vi "EX PROJ - Rotating Laptop Stand.vi"() -> ()   [LabVIEW 2018]
uses:
  <vilib>/Analysis/baseanly.llb/Mean (DBL).vi
  <vilib>/Analysis/NI_AALBase.lvlib
panel:
  out "offset":dbl
  out "power":dbl
  out "picture":picture
  in  "stop 2":bool
  out "fps":dbl
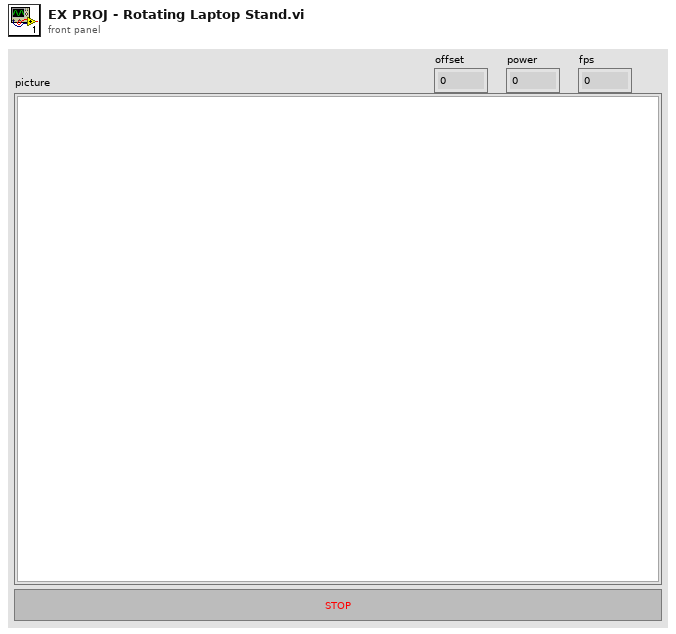
[diagram p1: front panel]
types:
  T1 = typedef "imagedata.ctl" = cluster{"image type":i32, "image depth":i32, "image":u8[], "mask":u8[], "colors":u32[], "Rectangle":cluster{"left":i16, "top":i16, "right":i16, "bottom":i16}}
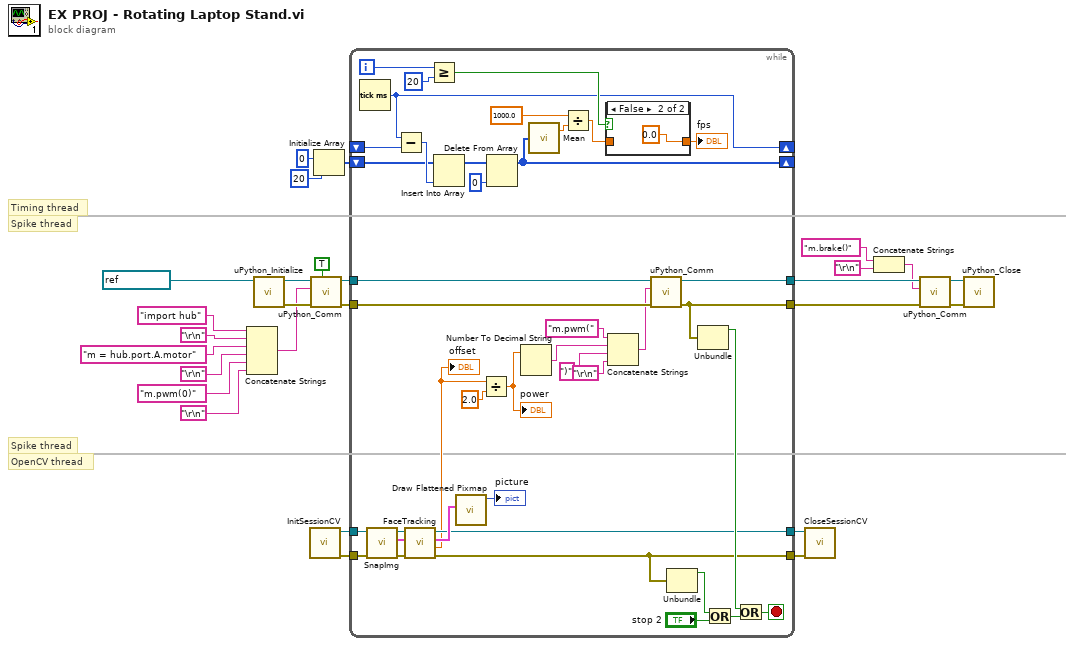
[diagram p0: block diagram]
diagram:
  # "Spike thread"
  # "OpenCV thread"
  # "Timing thread"
  # "Spike thread"
  n1 = Concatenate Strings("import hub" ("Script"), "\r\n", "m = hub.port.A.motor" ("Script"), "\r\n", "m.pwm(0)" ("Script"), "\r\n") -> (w11:string)
  n2 = call <userlib>:"uPython_Initialize.vi"("VISA Refnum in"=refnum<visa-resource-name> "COM15") -> ("error out"=w20:errorcluster, "VISA Refnum out"=w19:refnum<visa-resource-name>)  [unwired: 9 in]
  n3 = call "InitSessionCV.vi"() -> ("session out"=w24:refnum<k35>, "error out"=w23:errorcluster)  [unwired: 3 in]
  n4 = call <userlib>:"uPython_Comm.vi"("Wait for Reply?"=TRUE, "error in (no error)"=w20, "Script"=w11, "VISA Refnum in"=w19) -> ("error out"=w21:errorcluster, "VISA out"=w22:refnum<visa-resource-name>)  [unwired: 3 in, 3 out]
  n5 = Initialize Array(0, 20 ("dimension size")) -> (w25:i32[])
  n6 = while {
    shift-right: [w57] -> _
    shift-left: w25 -> [w58]
    shift-right: [w56] -> _
    shift-left: _ -> [w55]
    tunnel: w24 -> [w52]
    tunnel: w23 -> [w51]
    tunnel: w22 -> [w49]
    tunnel: w21 -> [w48]
    tunnel: [w47] -> w8
    tunnel: [w46] -> w7
    tunnel: [w32] -> w2
    tunnel: [w31] -> w1
    i -> [w54]
    stop <- w44 stop-if-true
    n7 = Tick Count (ms)() -> (millisecond timer value=w56:u32)
    n8 = call "SnapImg.vi"("error in (no error)"=w51, "session in"=w52) -> ("error out"=w35:errorcluster, "img out"=w36:T1, "session out"=w37:refnum<k35>)  [unwired: 3 in]
    n9 = Subtract(x=w56, y=w55) -> (x-y=w67:u32)
    n10 = call "FaceTracking.vi"("error in (no error)"=w35, "img in"=w36, "session in"=w37) -> ("error out"=w31:errorcluster, "offset from center"=w30:dbl, "img out"=w33:T1, "session out"=w32:refnum<k35>)  [unwired: 5 in]
    "offset" <- w30
    n11 = Greater Or Equal?(x=w54, y=20) -> (x >= y?=w59:bool)
    n12 = Insert Into Array(array=w58, new element=w67) -> (w66:i32[])  [unwired: 1 in]
    n13 = call <vilib>:"Draw Flattened Pixmap.vi"("image data"=w33) -> ("new picture"=→"picture":picture)  [unwired: 8 in]
    n14 = Divide(x=w30, y=2.0) -> (x/y=w28:dbl)
    "power" <- w28
    n15 = Delete From Array(array=w66, index=0) -> (array with subset deleted=w57:i32[])  [unwired: 1 in, 1 out]
    n16 = Number To Decimal String(number=w28) -> (decimal integer string=w39:string)  [unwired: 1 in]
    n17 = call-poly <vilib>:"Mean.vi"("X"=w57) -> ("mean"=w64:dbl)  [unwired: 1 out]
    n18 = Divide(x=1000.0 ("y"), y=w64) -> (x/y=w62:dbl)
    n19 = case shown="False" w59 {
      tunnel: w62 -> [w68 _]
      tunnel: [w68 0.0] -> w61
      frame True {
      }
      frame False {
      }
    }
    "fps" <- w61
    n20 = Concatenate Strings("m.pwm(" ("Script"), w39, ")" ("Script"), "\r\n") -> (w38:string)
    n21 = call <userlib>:"uPython_Comm.vi"("error in (no error)"=w48, "Script"=w38, "VISA Refnum in"=w49) -> ("error out"=w46:errorcluster, "VISA out"=w47:refnum<visa-resource-name>)  [unwired: 4 in, 3 out]
    n22 = Unbundle(w31) -> ("status"=w34:bool)  [unwired: 2 out]
    n23 = Unbundle(w46) -> ("status"=w43:bool)  [unwired: 2 out]
    n24 = Or(x=w34, y="stop 2") -> (x .or. y?=w45:bool)
    n25 = Or(x=w43, y=w45) -> (x .or. y?=w44:bool)
  }
  n26 = call "CloseSessionCV.vi"("error in (no error)"=w1, "Refnum in"=w2) -> ()  [unwired: 2 in]
  n27 = Concatenate Strings("m.brake()" ("Script"), "\r\n") -> (w6:string)
  n28 = call <userlib>:"uPython_Comm.vi"("error in (no error)"=w7, "Script"=w6, "VISA Refnum in"=w8) -> ("error out"=w9:errorcluster, "VISA out"=w10:refnum<visa-resource-name>)  [unwired: 4 in, 3 out]
  n29 = call <userlib>:"uPython_Close.vi"("error in"=w9, "VISA  in"=w10) -> ()  [unwired: 8 in, 2 out]
